vi "SMV.vi"(0 "System no.":i32=1 min=1 max=4 step=1, 2 "Axes to move":string[](array[string]), 3 "Commanded Steps":dbl[](array[numeric]) format="%.6f", 5 "error in":errorcluster) -> (19 "error out":errorcluster)   [LabVIEW 2020]
doc: "SMV (Start Step Motion)\n\nDescription\nSets the number and direction of the steps to be moved for the specified axes and starts the \nexecution of the steps.\nAll axes specified in the command start the motion simultaneously.\nDuring motion, a new SMV command sets the number and direction of steps to a new value; \nthe counting of the steps thus starts again from the beginning.\n\nFormat\nSMV{ <AxisID> <NumberOfSteps>}\nArguments\n<AxisID>\nAn axis of the controller\nThe available axes can be queried with USG? SYS. The axes for which the command is permitted \ncan be queried with USG? CMD SMV.\nPossible values: Alias of the axis (p. 94) \n<NumberOfSteps>\nNumber and direction of the steps to be moved\nThe data format is float.\nThe sign specifies the direction of motion.\nPossible values: Dependent on the controller\n\nResponse\nnone\n\nExample\nExample for SMV, SMV? (p. 59) and SMR? (p. 55): \n>>eax?\n<<AXIS_1=0\n<<AXIS_2=0\n<<AXIS_3=0\n>>eax axis_1 1\n>>eax axis_2 1\n>>eax axis_3 1\n>>eax?\n<<AXIS_1=1\n<<AXIS_2=1\n<<AXIS_3=1\n>>sam?\n<<AXIS_1=0x0\n<<AXIS_2=0x0\n<<AXIS_3=0x0\n>>frf\n>>frf?\n<<AXIS_1=1\n<<AXIS_2=1\n<<AXIS_3=1\n>>sam axis_3 0x7\n>>sam?\n<<AXIS_1=0x0\n<<AXIS_2=0x0\n<<AXIS_3=0x7\n>>pos?\n<<AXIS_1=2.507884837962963\n<<AXIS_2=-1.300802951388889\n<<AXIS_3=-8.426513671875E-3\n>>smv axis_3 5000\n>>smv?\n<<AXIS_3=5000.0\n>>smr?\n<<AXIS_3=4351.0\n>>smv?\n<<AXIS_3=5000.0\n>>smr?\n<<AXIS_3=2228.0\n>>pos?\n<<AXIS_1=2.507884837962963\n<<AXIS_2=-1.300802951388889\n<<AXIS_3=3.583245849609375\n>>smr?\n<<AXIS_3=351.0\n>>smr?\n<<AXIS_3=0\n>>pos?\n<<AXIS_1=2.507884837962963\n<<AXIS_2=-1.300802951388889\n<<AXIS_3=4.741072998046875\n>>pos?\n<<AXIS_1=2.507884837962963\n<<AXIS_2=-1.300802951388889\n<<AXIS_3=4.741072998046875\n\nNotes\nMotion is only executed if the following conditions are fulfilled for all specified axes: \n- The axis is in the Operation enabled state.\n- The mode of operation is set to 0x7.\nFor further details, see \"Drive State Machine\" (p. 101) and the status register of the axis (p. 97). \nThe STV? command (p. 66) queries the status register.\nThe SMV command starts a motion and thus sets bit 18 \"In Motion\" of the status register. \nThe SMV? command queries the number and direction of the commanded steps.\nThe SMR? command queries the current number and direction of the steps still to be moved.\nMotion can be stopped with the STP (p. 65) and HLT (p. 19) commands.\nFor further information, see \"Motion Behavior - GCS 3.0\" (p. 101). \n\nUser command level\nUSR"
panel:
  # "SMV (Start Step Motion)\n\nSets the number and direction of the steps to be moved for the specified axes and starts the execution of the steps.\nAll axes specified in the command start the motion simultaneously.\nDuring motion, a new SMV command sets the number and direction of steps to a new value; the counting of the steps thus starts again from the beginning."
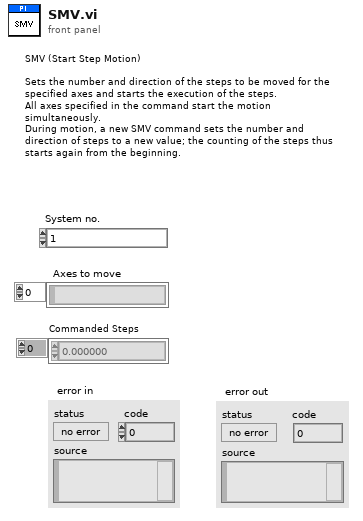
[diagram p1: front panel]
types:
  T1 = typedef "Syntax.ctl" = enum16{"GCS 1.0", "GCS 2.0", "GCS 3.0"}
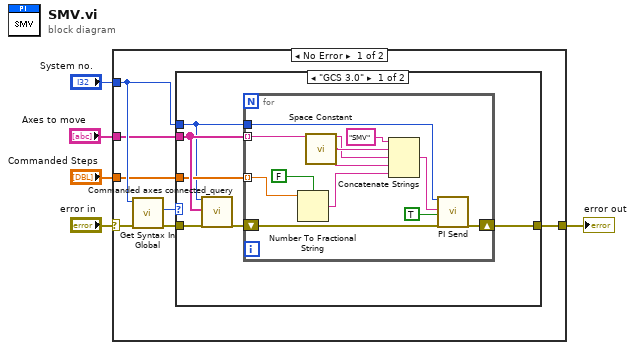
[diagram p0: block diagram]
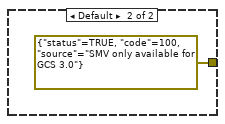
[diagram p2: hidden frame]
diagram:
  n1 = case shown="No Error" "error in" {
    selector: "error in" -> [w10 w31]
    tunnel: [w9 w31] -> w5
    tunnel: "Axes to move" -> [w7 _]
    tunnel: "System no." -> [w8 _]
    tunnel: "Commanded Steps" -> [w6 _]
    frame No Error {
      n2 = call "Get Syntax In Global.vi"("error in"=w10, "System no."=w8) -> ("error out"=w11:errorcluster, "Syntax"=w12:T1)  [unwired: 8 in]
      n3 = case shown="\"GCS 3.0\"" w12 {
        tunnel: [w14 errorcluster {"status"=TRUE, "code"=100, "source"="SMV only available for GCS 3.0"} ("error out")] -> w9
        tunnel: w11 -> [w17 _]
        tunnel: w8 -> [w13 _]
        tunnel: w7 -> [w16 _]
        tunnel: w6 -> [w15 _]
        frame "GCS 3.0" {
          n4 = call "Commanded axes connected_query.vi"("System no."=w13, "Commanded axes"=w16, "error in"=w17) -> ("error out"=w18:errorcluster)  [unwired: 16 out]
          n5 = for {
            shift-right: [w29] -> w14
            shift-left: w18 -> [w28]
            tunnel: w16 -> [w23] mode=indexing
            tunnel: w15 -> [w20] mode=indexing
            tunnel: w13 -> [w19]
            n6 = Number To Fractional String(use system decimal point (T)=FALSE, number=w20) -> (F-format string=w21:string)  [unwired: 2 in]
            n7 = call "Space Constant.vi"() -> ("String"=w24:string)
            n8 = Concatenate Strings("SMV", w24, w23, w24, w21) -> (w25:string)
            n9 = call "PI Send.vi"("System no."=w19, "String to send"=w25, "Attach termination char.?"=TRUE ("Attach Linefeed?"), "error in"=w28) -> ("error out"=w29:errorcluster)  [unwired: 2 in, 13 out]
          }
        }
        frame Default {
        }
      }
    }
    frame Error {
    }
  }
  "error out" <- w5
